vi "Test.vi"() -> ()   [LabVIEW 2022 SP3, in "LabSSH.lvlib"]
doc: "<License>This software is distributed under the BSD 3-Clause License. For the full license please see license.txt or visit www.labvolution.com/license</License>"
uses:
  LabSSH.lvlib
  Connection Info..cluster.ctl
  Password..cluster.ctl
  Private Public Key..cluster.ctl
  <vilib>/Utility/miscctls.llb/LVForegroundBackgroundColorsTypeDef.ctl
  connect_password.vi
  connect_key.vi
panel:
  in  "Connection Name":string
  in  "Close":bool
  in  "Connect":bool
  in  "Expected Response":string
  in  "Private_Public Key":T1
  in  "Connection Type":enum16{"Password", "Private Key"}(ring)
  out "Method Response":string
  in  "error in (no error)":errorcluster
  out "isSshConnected":bool
  in  "Password":T2
  in  "Connection Info.":T3={"Remote"="", "Username"="", "Port (22)"=22}
  out "Output":string
  # "http://www.labvolution.com/blog/"
  # "C:\\\\Working Folder\\\\ssh.git\\\\LabSSH\\\\raspberrypi_private_openssh.ppk"
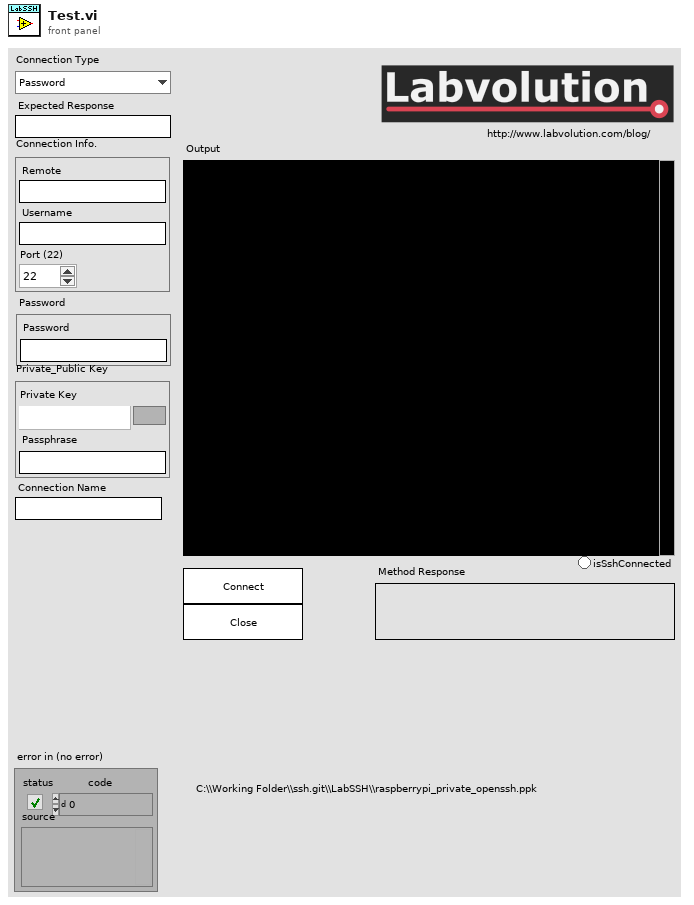
[diagram p1: front panel]
types:
  T1 = typedef "LabSSH.lvlib/Private Public Key..cluster.ctl" = cluster{"Private Key":path, "Passphrase":string}
  T2 = typedef "LabSSH.lvlib/Password..cluster.ctl" = cluster{"Password":string}
  T3 = typedef "LabSSH.lvlib/Connection Info..cluster.ctl" = cluster{"Remote":string, "Username":string, "Port (22)":i32}
  T4 = typedef "LVForegroundBackgroundColorsTypeDef.ctl" = cluster{"Foreground Color":u32, "Background Color":u32}
  T5 = enum32{"invalid app kind", "Development System", "Run Time System", "Student Edition", "Embedded LabVIEW", "Evaluation", "Custom"}
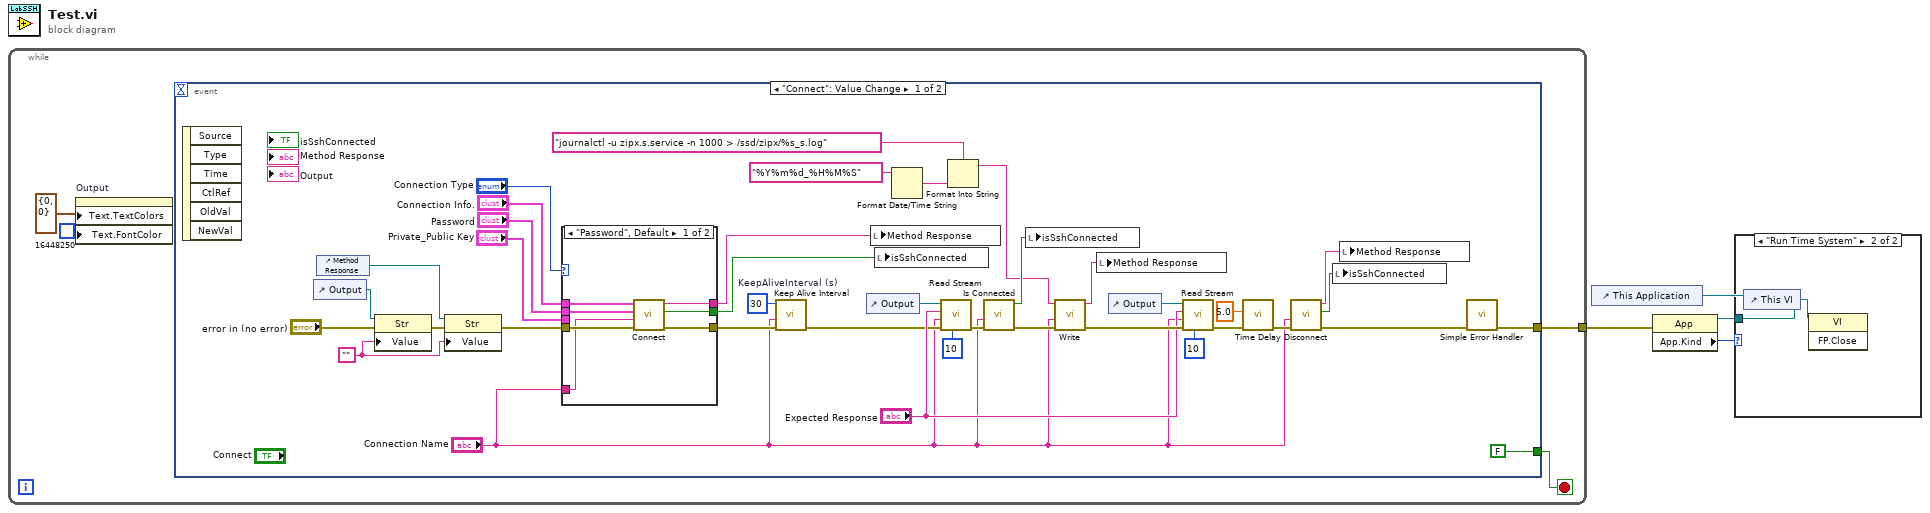
[diagram p0: block diagram]
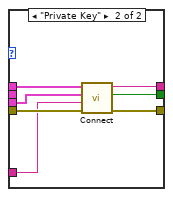
[diagram p2: hidden frame]
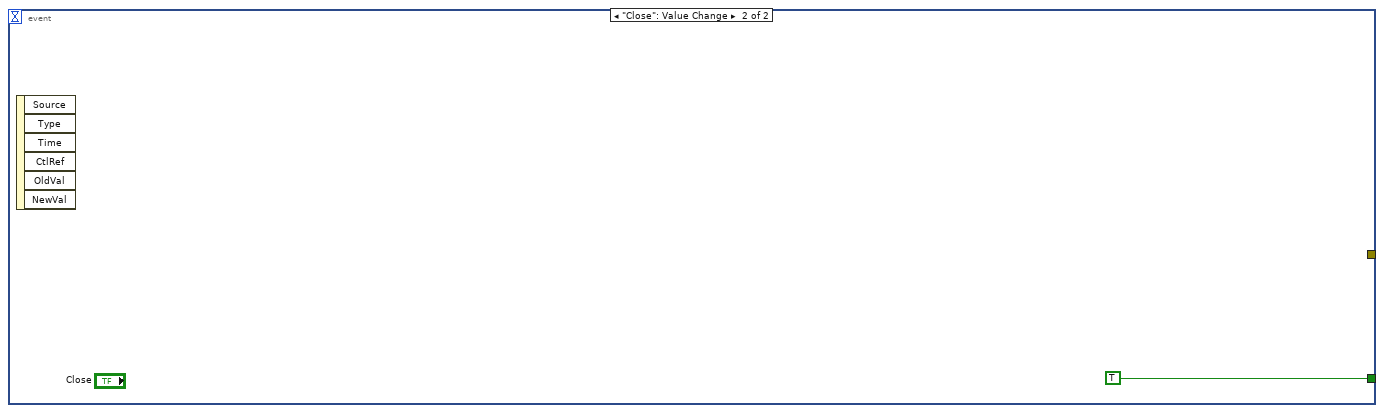
[diagram p3: hidden frame]
diagram:
  n1 = while {
    tunnel: [w5] -> w3
    stop <- w8 stop-if-true
    n2 = property on="Output" class="Str"("Text.TextColors"=T4 {"Foreground Color"=0, "Background Color"=0} ("Text.Colors"), "Text.FontColor"=u32 16448250 ("Text.Colors:BG Color")) -> ()  [unwired: 2 in, 2 out]
    n3 = event shown="[0] \"Connect\": Value Change" {
      selector: _ -> [_ _]
      dyn-events: _ -> [_ _]
      timeout: _ -> [_ _]
      tunnel: [FALSE TRUE] -> w8
      tunnel: [w19 _] -> w5
      event "Connect": Value Change {
        w15 = 30  # KeepAliveInterval (s)
        w27 = ""
        n4 = event-data() -> ()  [unwired: 1 in, 6 out]
        n5 = control-ref of="Output"() -> (w30:refnum<vi>)
        n6 = control-ref of="Method Response"() -> (w28:refnum<vi>)
        n7 = property class="Str"(reference=w30, error in="error in (no error)", "Value"=w27) -> (error out=w31:errorcluster)  [unwired: 1 out]
        n8 = property class="Str"(reference=w28, error in=w31, "Value"=w27) -> (error out=w29:errorcluster)  [unwired: 1 out]
        n9 = case shown="\"Password\", Default" "Connection Type" {
          tunnel: [w53 w58] -> w17
          tunnel: "Connection Info." -> [w52 w60]
          tunnel: "Password" -> [w51 _]
          tunnel: [w50 w57] -> w40
          tunnel: [w49 w56] -> w34
          tunnel: w29 -> [w48 w59]
          tunnel: "Private_Public Key" -> [_ w55]
          tunnel: "Connection Name" -> [w47 w54]
          frame "Password", Default {
            n10 = call-poly "Connect.vi"("error in (no error)"=w48, "Connection Name"=w47, "Password"=w51, "Connection Info."=w52) -> ("error out"=w53:errorcluster, "isSshConnected"=w50:bool, "Return String"=w49:string)  [unwired: 5 in]
          }
          frame "Private Key" {
            n11 = call-poly "Connect.vi"("error in (no error)"=w59, "Connection Name"=w54, "Private_Public Key"=w55, "Connection Info."=w60) -> ("error out"=w58:errorcluster, "isSshConnected"=w57:bool, "Return String"=w56:string)  [unwired: 5 in]
          }
        }
        n12 = call "Keep Alive Interval.vi"("error in (no error)"=w17, "Connection Name"="Connection Name", "KeepAliveInterval (s)"=w15) -> ("error out"=w18:errorcluster)  [unwired: 8 in]
        n13 = control-ref of="Output"() -> (w45:refnum<vi>)
        n14 = local write "Method Response"(w34) -> ()
        n15 = local write "isSshConnected"(w40) -> ()
        n16 = Format Date/Time String(time format string (%c)="%Y%m%d_%H%M%S") -> (date/time string=w12:string)  [unwired: 2 in]
        n17 = call "Read Stream.vi"("Timout (s)"=10, "error in (no error)"=w18, "Connection Name"="Connection Name", "Expected Response"="Expected Response", "Output ref"=w45) -> ("error out"=w41:errorcluster)  [unwired: 6 in]
        n18 = Format Into String(format string="journalctl -u zipx.s.service -n 1000 > /ssd/zipx/%s_s.log" ("Command"), w12) -> (resulting string=w9:string)  [unwired: 2 in, 1 out]
        n19 = call "Is Connected.vi"("error in (no error)"=w41, "Connection Name"="Connection Name") -> ("error out"=w38:errorcluster, "isSshConnected"=w39:bool)  [unwired: 8 in]
        n20 = local write "isSshConnected"(w39) -> ()
        n21 = call "Write.vi"("error in (no error)"=w38, "Connection Name"="Connection Name", "Command"=w9) -> ("error out"=w35:errorcluster, "Return String"=w33:string)  [unwired: 7 in]
        n22 = local write "Method Response"(w33) -> ()
        n23 = control-ref of="Output"() -> (w37:refnum<vi>)
        n24 = call "Read Stream.vi"("Timout (s)"=10, "error in (no error)"=w35, "Connection Name"="Connection Name", "Expected Response"="Expected Response", "Output ref"=w37) -> ("error out"=w22:errorcluster)  [unwired: 6 in]
        n25 = call "Time Delay"("error in (no error)"=w22, "Delay Time (s)"=5.0) -> ("error out"=w21:errorcluster)  [unwired: 9 in]
        n26 = call "Disconnect.vi"("error in (no error)"=w21, "Connection Name"="Connection Name") -> ("error out"=w32:errorcluster, "isSshConnected"=w13:bool, "Return String"=w14:string)  [unwired: 7 in]
        n27 = local write "isSshConnected"(w13) -> ()
        n28 = local write "Method Response"(w14) -> ()
        n29 = call <vilib>:"Simple Error Handler.vi"("error in (no error)"=w32) -> ("error out"=w19:errorcluster)  [unwired: 4 in, 4 out]
      }
      event "Close": Value Change {
        n30 = event-data() -> ()  [unwired: 1 in, 6 out]
      }
    }
  }
  n31 = control-ref of="This Application"() -> (w4:refnum<vi>)
  n32 = property class="App"(reference=w4, error in=w3) -> (reference out=w1:refnum<vi>, "App.Kind"=w2:T5)  [unwired: 1 out]
  n33 = case shown="\"Run Time System\"" w2 {
    tunnel: w1 -> [_ _]
    frame "invalid app kind", Default {
    }
    frame "Run Time System" {
      n34 = control-ref of="This VI"() -> (w62:refnum<vi>)
      n35 = invoke class="VI" method="FP.Close"(reference=w62) -> ()  [unwired: 2 in, 3 out]
    }
  }
